vi "EOL Check Abort Test Prerun.vi"(8 "Next State":string, 10 "Abort Test":bool, 11 "Test Running?":bool) -> (1 "State":string)   [LabVIEW 2018]
uses:
  05.UserVI's/type defs/EOL Global Digital Input Control.ctl
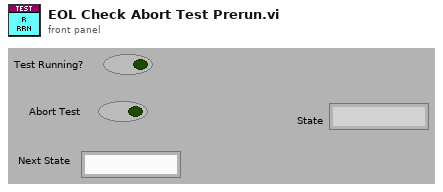
[diagram p1: front panel]
types:
  T1 = typedef "EOL Global Digital Input Control.ctl" = enum16{"Dev2/port0/line0", "Dev2/port0/line1", "Dev2/port0/line2", "Dev2/port0/line3", "Dev2/port0/line4", "Dev2/port0/line5", "Dev2/port0/line6", "Dev2/port0/line7", "Dev2/port1/line0", "Dev2/port1/line1", "Dev2/port1/line2", "Dev2/port1/line3", "Dev2/port1/line4", "Dev2/port1/line5", "Dev2/port1/line6", "Dev2/port1/line7", "Dev2/port2/line0", "Dev2/port2/line1", "Dev2/port2/line2", "Dev2/port2/line3", "Dev2/port2/line4", "Dev2/port2/line5", "Dev2/port2/line6", "Dev2/port2/line7", "Prerun Start Test", "Prerun Abort Test", "Audit Start Test", "Audit Abort Test", "Dev2/port3/line4", "Dev2/port3/line5", "Breakin Start Test", "Breakin Abort Test", "Not Implemented"}
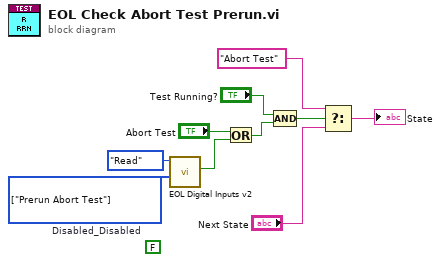
[diagram p0: block diagram]
diagram:
  (unwired) FALSE  # Disabled_Disabled
  w2 = T1[] [enum."Prerun Abort Test"] items=["Dev2/port0/line0", "Dev2/port0/line1", "Dev2/port0/line2", "Dev2/port0/line3", "Dev2/port0/line4", "Dev2/port0/line5", "Dev2/port0/line6", "Dev2/port0/line7", "Dev2/port1/line0", "Dev2/port1/line1", "Dev2/port1/line2", "Dev2/port1/line3", "Dev2/port1/line4", "Dev2/port1/line5", "Dev2/port1/line6", "Dev2/port1/line7", "Dev2/port2/line0", "Dev2/port2/line1", "Dev2/port2/line2", "Dev2/port2/line3", "Dev2/port2/line4", "Dev2/port2/line5", "Dev2/port2/line6", "Dev2/port2/line7", "Prerun Start Test", "Prerun Abort Test", "Audit Start Test", "Audit Abort Test", "Dev2/port3/line4", "Dev2/port3/line5", "Breakin Start Test", "Breakin Abort Test", "Not Implemented"] ("Digital Inputs Array")
  n1 = call "EOL Digital Inputs v2.vi"("Digital Inputs Array"=w2, "Mode"=enum16{"Init", "Read", "Read All", "Close"}."Read") -> ("Single Input"=w1:bool)  [unwired: 7 in, 2 out]
  n2 = Or(x="Abort Test", y=w1) -> (x .or. y?=w4:bool)
  n3 = Compound Arithmetic op=AND("Test Running?", w4) -> (w7:bool)
  n4 = Select(t="Abort Test", s=w7, f="Next State") -> (s? t:f=→"State":string)
